vi "Double move fwd PID.vi"(4 "Time to stop":i32=300, 5 "Range":cluster{"output high":dbl, "output low":dbl}={"output high"=1.0, "output low"=0.0} {"output low" format="%.2f"; "output high" format="%.2f"}, 6 "Loop Timer":i32=20, 7 "Gains":T1={"proportional gain (Kc)"=1.0, "integral time (Ti, min)"=0.01, "derivative time (Td, min)"=0.0} {"derivative time (Td, min)" format="%.3f"; "integral time (Ti, min)" format="%.3f"; "proportional gain (Kc)" format="%.3f"}, 8 "Precision":dbl=0.5 format="%#_13g", 9 "Encoder Right":dbl, 10 "Encoder Left":dbl, 11 "Distance":dbl) -> (0 "Both finished?":bool, 2 "PWM Right":dbl=0.5 format="%#_13g", 3 "PWM Left":dbl=0.5 format="%#_13g")   [LabVIEW 2017]
panel:
  # "Time to stop - Tempo que o encoder deve retornar um valor dentro do range da precision para a função considerar que o sistema está parado.\n\nDistance - Setpoint em unidades do encoder.\n\nLoop Timer - Tempo de iteração do loop em que a função está.\n\nPrecision - Range que a função considera \"close enough\" ao setpoint.\n\nEncoder Right - Valor atual do encoder da direita.\n\nEncoder Left - Valor atual do encoder da esquerda\n\nRate limit - Limite de aceleração/desaceleração do sistema.\n\nGains - Ganhos do PID.\n\nRange - limite superior e inferior do PID.\n\nSoft Start - constante que aumenta ou diminui o tempo de aceleração no início do movimento"
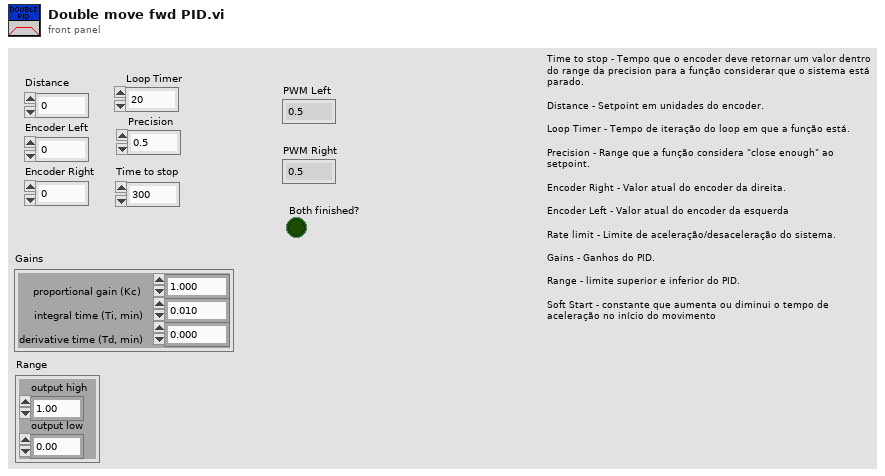
[diagram p1: front panel]
types:
  T1 = cluster{"proportional gain (Kc)":dbl, "integral time (Ti, min)":dbl, "derivative time (Td, min)":dbl}
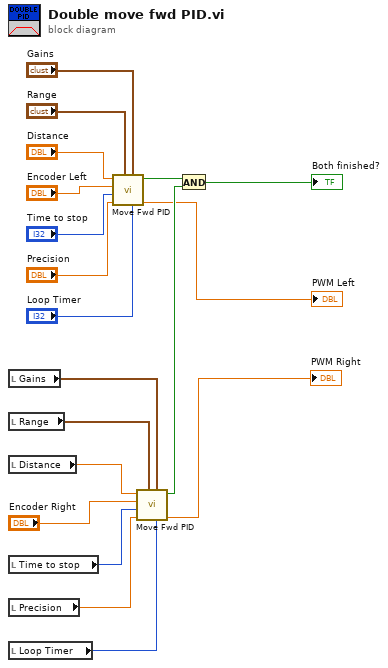
[diagram p0: block diagram]
diagram:
  n1 = local read "Gains"() -> (w11:T1)
  n2 = local read "Range"() -> (w10:cluster{"output high":dbl, "output low":dbl})
  n3 = local read "Distance"() -> (w9:dbl)
  n4 = local read "Time to stop"() -> (w8:i32)
  n5 = local read "Precision"() -> (w7:dbl)
  n6 = local read "Loop Timer"() -> (w6:i32)
  n7 = call "Move Fwd PID.vi"("Loop Timer"="Loop Timer", "Gains"="Gains", "Range"="Range", "Precision"="Precision", "Time to stop"="Time to stop", "Encoder Count"="Encoder Left", "Distance"="Distance") -> ("Output"=→"PWM Left":dbl, "Finished?"=w5:bool)  [unwired: 3 in]
  n8 = call "Move Fwd PID.vi"("Loop Timer"=w6, "Gains"=w11, "Range"=w10, "Precision"=w7, "Time to stop"=w8, "Encoder Count"="Encoder Right", "Distance"=w9) -> ("Output"=→"PWM Right":dbl, "Finished?"=w4:bool)  [unwired: 3 in]
  n9 = And(x=w5, y=w4) -> (x .and. y?=→"Both finished?":bool)
